vi "Initialize camera.vi"(11 "Session In":T1="cam0") -> (0 "error out":errorcluster, 3 "Session Out":T1)   [LabVIEW 2018]
uses:
  <vilib>/userdefined/High Color/IMAQdx.ctl
  <vilib>/vision/driver/NI_Vision_Acquisition_Software.lvlib
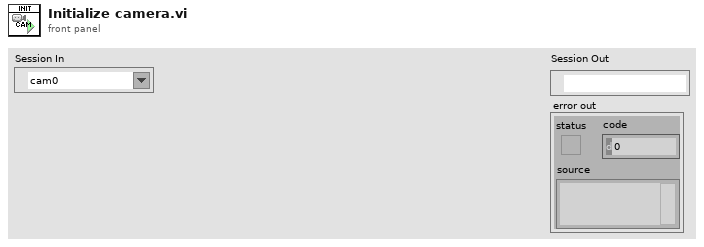
[diagram p1: front panel]
types:
  T1 = typedef "IMAQdx.ctl" = refnum<k21>
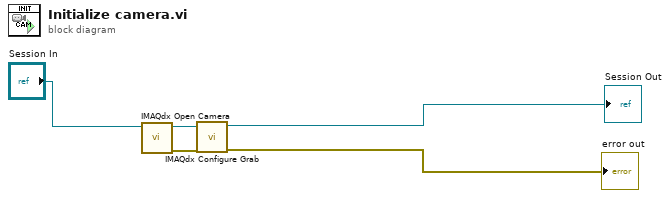
[diagram p0: block diagram]
diagram:
  n1 = call <vilib>:"IMAQdx Open Camera.vi"("Session In"="Session In") -> ("error out"=w4:errorcluster, "Session Out"=w5:T1)  [unwired: 9 in]
  n2 = call <vilib>:"IMAQdx Configure Grab.vi"("error in"=w4, "Session In"=w5) -> ("error out"=→"error out":errorcluster, "Session Out"=→"Session Out":T1)  [unwired: 8 in]
